vi "Delay.vi"(8 "error in (no error)":errorcluster, 9 "Delay":u32) -> (0 "error out":errorcluster)   [LabVIEW 2017]
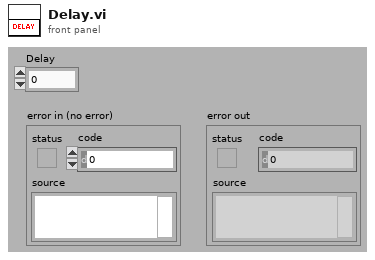
[diagram p1: front panel]
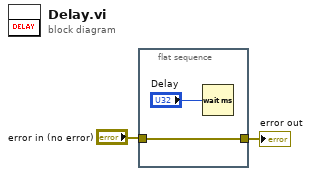
[diagram p0: block diagram]
diagram:
  n1 = flat-sequence {
    tunnel: [w4] -> w2
    tunnel: "error in (no error)" -> [w4]
    frame #0 {
      n2 = Wait (ms)(milliseconds to wait="Delay") -> ()  [unwired: 1 out]
    }
  }
  "error out" <- w2
